vi "flip.vi"(8 "error in (no error)":errorcluster, 10 "Type of Symmetry":u32(ring) items=["Horizontal", "Vertical", "Central", "1st Diagonal", "2nd Diagonal"], 11 "Image in":refnum<class "Image.lvclass">) -> (0 "error out":errorcluster, 3 "Image out":refnum<class "Image.lvclass">)   [LabVIEW 2010, in "Image.lvclass"]
uses:
  Image.lvclass
  storage_mode.ctl
  ErrorController/ErrorController/class_data.vi
  <vilib>/vision/NI_Vision_Development_Module.lvlib
  ErrorController/ErrorController/ErrorController.lvclass
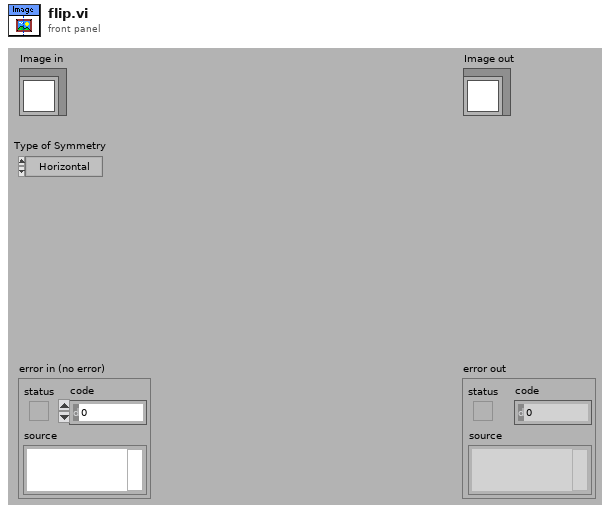
[diagram p1: front panel]
types:
  T1 = typedef "Image.lvclass/storage_mode.ctl" = enum16{"RAM", "disk"}
  T2 = typedef "IMAQ Image.ctl" = refnum<image>
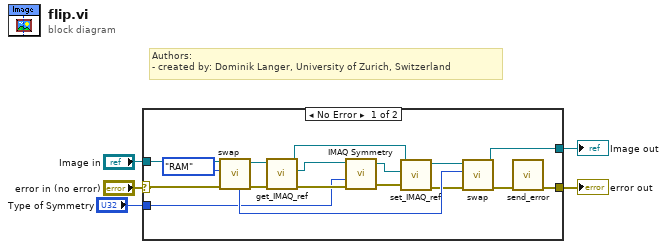
[diagram p0: block diagram]
diagram:
  # "Authors: \n- created by: Dominik Langer, University of Zurich, Switzerland"
  n1 = case shown="No Error" "error in (no error)" {
    selector: "error in (no error)" -> [w15 w24]
    tunnel: [w6 w24] -> w4
    tunnel: [w10 w23] -> w2
    tunnel: "Image in" -> [w11 w23]
    tunnel: "Type of Symmetry" -> [w8 _]
    frame No Error {
      n2 = call-dynamic "swap.vi"("error in (no error)"=w15, "storage type target"=storage_mode."RAM", "Image in"=w11) -> ("error out"=w20:errorcluster, "Image out"=w19:refnum<class "Image.lvclass">, "previous storage mode"=w21:T1)  [unwired: 6 out]
      n3 = call-dynamic "get_IMAQ_ref.vi"("error in (no error)"=w20, "Image.lvclass in"=w19) -> ("error out"=w14:errorcluster, "Image"=w13:T2, "Image.lvclass out"=w18:refnum<class "Image.lvclass">)  [unwired: 7 out]
      n4 = call "IMAQ Symmetry"("error in (no error)"=w14, "Type of Symmetry"=w8, "Image Src"=w13) -> ("error out"=w9:errorcluster, "Image Dst Out"=w12:T2)  [unwired: 1 in, 1 out]
      n5 = call-dynamic "set_IMAQ_ref.vi"("error in (no error)"=w9, "Image"=w12, "Image.lvclass in"=w18) -> ("error out"=w17:errorcluster, "Image.lvclass out"=w16:refnum<class "Image.lvclass">)  [unwired: 7 out]
      n6 = call-dynamic "swap.vi"("error in (no error)"=w17, "storage type target"=w21, "Image in"=w16) -> ("error out"=w7:errorcluster, "Image out"=w10:refnum<class "Image.lvclass">)  [unwired: 7 out]
      n7 = call "send_error.vi"("error in (no error)"=w7) -> ("error out"=w6:errorcluster)  [unwired: 10 in]
    }
    frame Error {
    }
  }
  "error out" <- w4
  "Image out" <- w2
